vi "DequeueEvent.vi"(8 "Error Input":errorcluster caption="Error In", 11 "Queue In":refnum<queue>) -> (0 "Error Output":errorcluster caption="Error Out", 2 "EventJson":string, 3 "Queue Out":refnum<queue>)   [LabVIEW 2017, in "LiteAgentSDK.lvlib"]
uses:
  LiteAgentSDK.lvlib
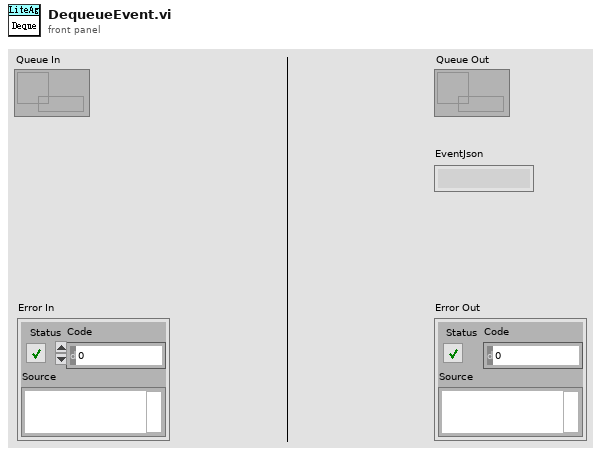
[diagram p1: front panel]
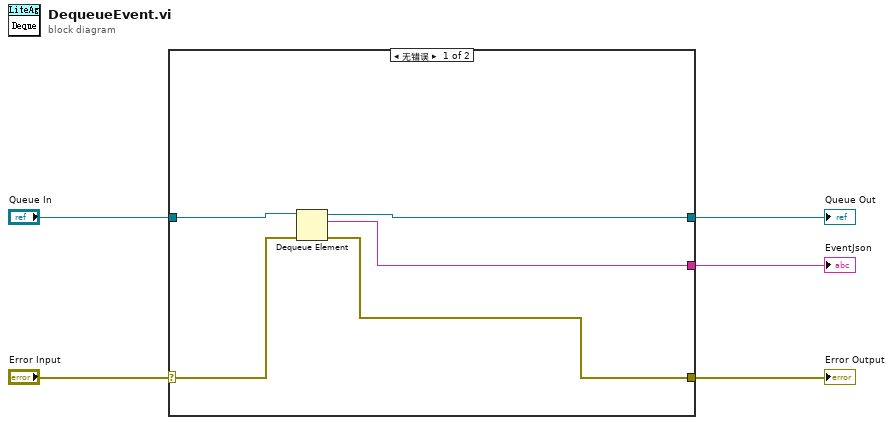
[diagram p0: block diagram]
diagram:
  n1 = case shown="无错误" "Error Input" {
    selector: "Error Input" -> [w9 w12]
    tunnel: [w6 w12] -> w4
    tunnel: "Queue In" -> [w10 w11]
    tunnel: [w8 w11] -> w2
    tunnel: [w7 _] -> w1
    frame No Error {
      n2 = Dequeue Element(queue=w10, error in (no error)=w9) -> (queue out=w8:refnum<queue>, element=w7:string, error out=w6:errorcluster)  [unwired: 1 in, 1 out]
    }
    frame Error {
    }
  }
  "Error Output" <- w4
  "EventJson" <- w1
  "Queue Out" <- w2
